vi "Desplazamientos_vrl.vi"(6 "Indice":u16, 8 "Rotacion":dbl[](array[numeric])=[1.0, 1.0, 1.0, 1.0], 9 "Translacion":dbl[](array[numeric])=[1.0, 1.0, 1.0], 10 "Escala":dbl[](array[numeric])=[1.0, 1.0, 1.0]) -> (3 "Salida":string[](array[string]))   [LabVIEW 2017]
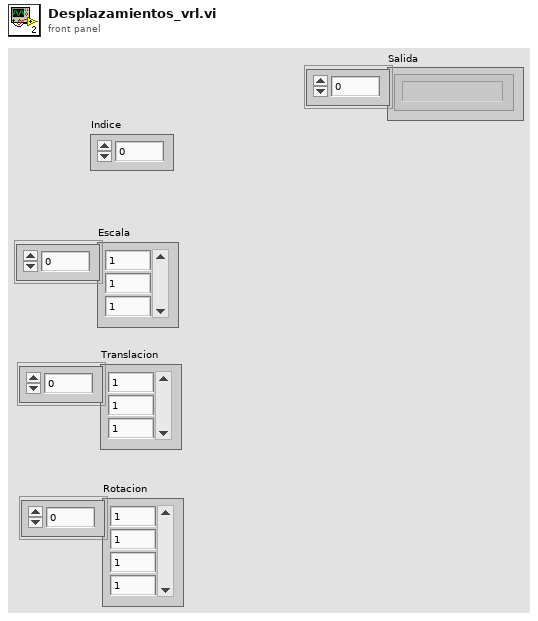
[diagram p1: front panel]
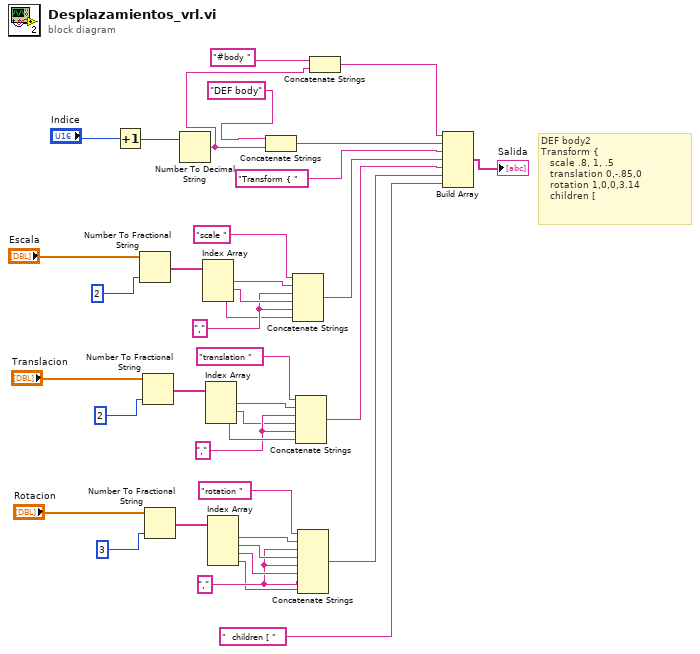
[diagram p0: block diagram]
diagram:
  w11 = ","
  w25 = ","
  w30 = ","
  # "DEF body2\nTransform { \n   scale .8, 1, .5\n   translation 0,-.85,0\n   rotation 1,0,0,3.14\n   children ["
  n1 = Increment(x="Indice") -> (x+1=w37:u16)
  n2 = Number To Fractional String(number="Escala", precision (6)=i16 2) -> (F-format string=w34:string[])  [unwired: 2 in]
  n3 = Number To Fractional String(number="Translacion", precision (6)=i16 2) -> (F-format string=w21:string[])  [unwired: 2 in]
  n4 = Number To Fractional String(number="Rotacion", precision (6)=i16 3) -> (F-format string=w16:string[])  [unwired: 2 in]
  n5 = Number To Decimal String(number=w37) -> (decimal integer string=w3:string)  [unwired: 1 in]
  n6 = Index Array(array=w34) -> (element #1=w32:string, element #2=w31:string, element #3=w29:string)  [unwired: 3 in]
  n7 = Index Array(array=w21) -> (element #1=w23:string, element #2=w24:string, element #3=w26:string)  [unwired: 3 in]
  n8 = Index Array(array=w16) -> (element #1=w14:string, element #2=w13:string, element #3=w12:string, element #4=w10:string)  [unwired: 4 in]
  n9 = Concatenate Strings("DEF body", w3) -> (w4:string)
  n10 = Concatenate Strings("scale ", w32, w30, w31, w30, w29) -> (w27:string)
  n11 = Concatenate Strings("translation ", w23, w25, w24, w25, w26) -> (w9:string)
  n12 = Concatenate Strings("rotation ", w14, w11, w13, w11, w12, w11, w10) -> (w8:string)
  n13 = Concatenate Strings("#body ", w3) -> (w1:string)
  n14 = Build Array(w1, w4, "Transform { ", w27, w9, w8, "  children [ ") -> (→"Salida":string[])
